vi "titration_data_accessor.vi"() -> ()   [LabVIEW 2010]
panel:
  in  "Sample Data":T1
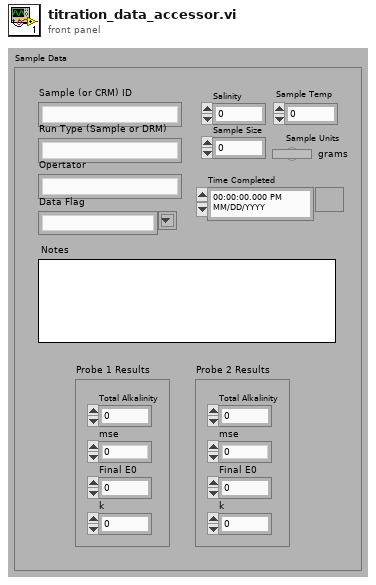
[diagram p1: front panel]
types:
  T1 = cluster{"Sample (or CRM) ID":string, "Run Type (Sample or DRM)":string, "Opertator":string, "Data Flag":string, "Salinity":dbl, "Sample Temp":dbl, "Sample Size":dbl, "Sample Units":bool, "Time Completed":timestamp, "Notes":string, "Probe 1 Results":cluster{"Total Alkalinity":dbl, "mse":dbl, "Final E0":dbl, "k":dbl}, "Probe 2 Results":cluster{"Total Alkalinity":dbl, "mse":dbl, "Final E0":dbl, "k":dbl}}
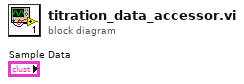
[diagram p0: block diagram]
diagram:
